vi "CMD_INC.vi"(6 "Gantry in":refnum<class "Gantry.lvclass">, 8 "error in (no error)":errorcluster, 10 "Arguments":string[](array[string]), 11 "gScript Interpreter in":refnum<class "gScript Interpreter.lvclass">) -> (0 "error out":errorcluster, 3 "gScript Interpreter out":refnum<class "gScript Interpreter.lvclass">, 4 "Gantry out":refnum<class "Gantry.lvclass">)   [LabVIEW 2024, in "gScript Interpreter.lvclass"]
uses:
  gScript Interpreter.lvclass
  Shared Components/Gantry Class/Gantry.lvclass
  Type Definitions/Memory Cell.ctl
  Type Definitions/Memory Cell Type Enum.ctl
  gScript Interpreter.lvclass/gScript Interpreter.ctl
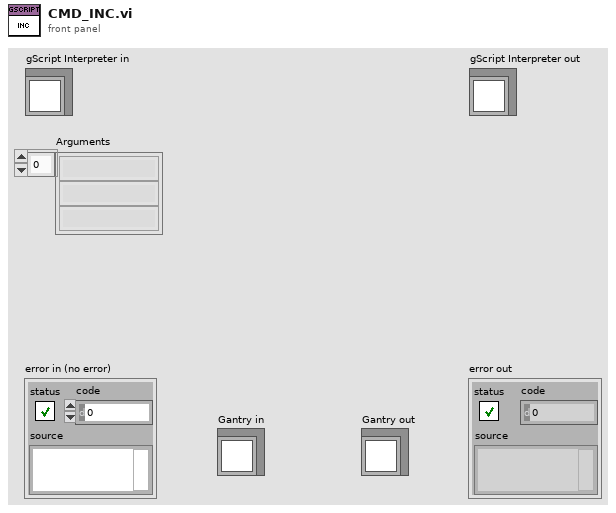
[diagram p1: front panel]
types:
  T1 = typedef "Memory Cell.ctl" = cluster{"type":T2, "x":dbl, "y":dbl, "z":dbl, "w":dbl}
  T2 = typedef "Memory Cell Type Enum.ctl" = enum16{"integer", "float", "vector", "rotation"}
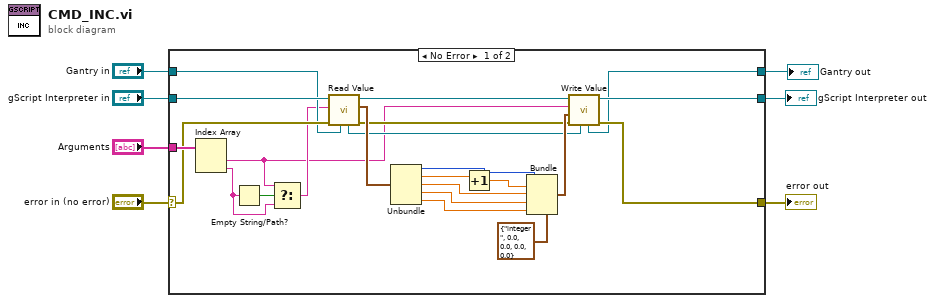
[diagram p0: block diagram]
diagram:
  n1 = case shown="No Error" "error in (no error)" {
    selector: "error in (no error)" -> [w20 w33]
    tunnel: [w23 w33] -> w6
    tunnel: [w24 w32] -> w4
    tunnel: "gScript Interpreter in" -> [w21 w32]
    tunnel: "Arguments" -> [w30 _]
    tunnel: "Gantry in" -> [w14 w31]
    tunnel: [w12 w31] -> w1
    frame No Error {
      n2 = Index Array(array=w30) -> (element #1=w9:string, element #2=w8:string)  [unwired: 2 in]
      n3 = Empty String/Path?(string/path=w8) -> (empty?=w11:bool)
      n4 = Select(t=w9, s=w11, f=w8) -> (s? t:f=w10:string)
      n5 = call-dynamic "Read Value.vi"("Gantry in"=w14, "error in (no error)"=w20, "String in"=w10, "gScript Interpreter in"=w21) -> ("error out"=w25:errorcluster, "Memory Cell"=w29:T1, "gScript Interpreter out"=w28:refnum<class "gScript Interpreter.lvclass">, "Gantry out"=w13:refnum<class "Gantry.lvclass">)  [unwired: 4 in]
      n6 = Unbundle(w29) -> ("type"=w22:T2, "x"=w19:dbl, "y"=w17:dbl, "z"=w16:dbl, "w"=w15:dbl)
      n7 = Increment(x=w19) -> (x+1=w18:dbl)
      n8 = Bundle(cluster=T1 {"type"=enum."integer", "x"=0.0, "y"=0.0, "z"=0.0, "w"=0.0} ("Memory Cell"), "type"=w22, "x"=w18, "y"=w17, "z"=w16, "w"=w15) -> (w26:T1)
      n9 = call-dynamic "Write Value.vi"("Gantry in"=w13, "error in (no error)"=w25, "Value"=w26, "Address"=w9, "gScript Interpreter in"=w28) -> ("error out"=w23:errorcluster, "gScript Interpreter out"=w24:refnum<class "gScript Interpreter.lvclass">, "Gantry out"=w12:refnum<class "Gantry.lvclass">)  [unwired: 4 in]
    }
    frame Error {
    }
  }
  "error out" <- w6
  "gScript Interpreter out" <- w4
  "Gantry out" <- w1
